vi "Change Time.vi"(8 "error in (no error)":errorcluster, 10 "Time":timestamp, 11 "VISA resource name":refnum<visa-resource-name>) -> (0 "error out":errorcluster, 3 "VISA resource name out":refnum<visa-resource-name>)   [LabVIEW 2017, in "Sefram DAS220.lvlib"]
doc: "Change the time of the device."
uses:
  <instrlib>/Sefram DAS220/Sefram DAS220.lvlib
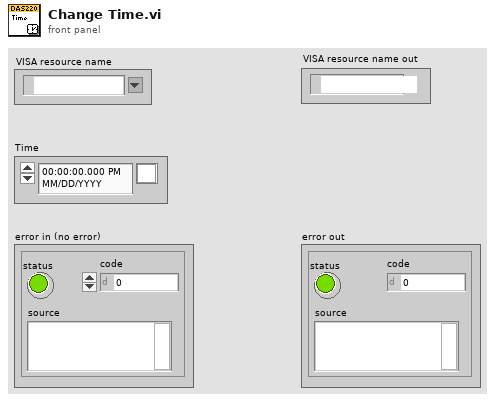
[diagram p1: front panel]
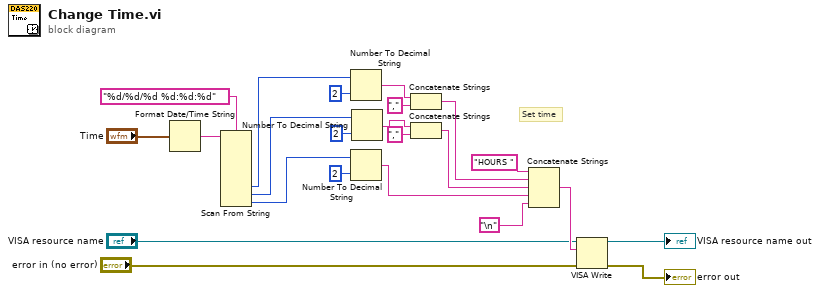
[diagram p0: block diagram]
diagram:
  # "Set time"
  n1 = Format Date/Time String(seconds (now)="Time") -> (date/time string=w5:string)  [unwired: 2 in]
  n2 = Scan From String(format string="%d/%d/%d %d:%d:%d", input string=w5) -> (output 4=w4:i32, output 5=w3:i32, output 6=w2:i32)  [unwired: 11 in, 3 out]
  n3 = Number To Decimal String(number=w4, width (-)=i16 2) -> (decimal integer string=w13:string)
  n4 = Number To Decimal String(number=w2, width (-)=i16 2) -> (decimal integer string=w7:string)
  n5 = Number To Decimal String(number=w3, width (-)=i16 2) -> (decimal integer string=w9:string)
  n6 = Concatenate Strings(w13, "," ("string")) -> (w11:string)
  n7 = Concatenate Strings(w9, "," ("string")) -> (w8:string)
  n8 = Concatenate Strings("HOURS " ("string"), w11, w8, w7, "\n") -> (w23:string)
  n9 = VISA Write(VISA resource name="VISA resource name", write buffer=w23, error in (no error)="error in (no error)") -> (VISA resource name out=→"VISA resource name out":refnum<visa-resource-name>, error out=→"error out":errorcluster)  [unwired: 1 out]
